vi "Periodic Tasks.vi"(8 "error in":errorcluster) -> ()   [LabVIEW 2017]
doc: "This VI runs in parallel to other robot code. It can contain as many user-defined periodic loops as you need. These can carry out PID or other sorts of timed response."
uses:
  <vilib>/Rock Robotics/WPI/Utilities/WPI_GetSetVariantRefNum.vi
  Robot Global Data.vi
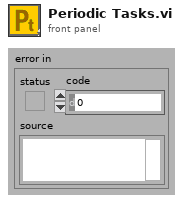
[diagram p1: front panel]
types:
  T1 = typedef "WPI_JoystickDevRef.ctl" = cluster{"Device":T2}
  T2 = typedef "WPI_JoystickDeviceEnum.ctl" = enum16{"USB 0", "USB 1", "USB 2", "USB 3", "USB 4", "USB 5"}
  T3 = typedef "WPI_SwitchDevRef.ctl" = cluster{"DevStatus":errorcluster, "DIO Channel":T4, "CntIndex":T5, "Normally Closed":bool}
  T4 = typedef "FPGA_DIOChannel.ctl" = enum8{"DIO 0", "DIO 1", "DIO 2", "DIO 3", "DIO 4", "DIO 5", "DIO 6", "DIO 7", "DIO 8", "DIO 9", "DIO MXP 0", "DIO MXP 1", "DIO MXP 2", "DIO MXP 3", "DIO MXP 4", "DIO MXP 5", "DIO MXP 6", "DIO MXP 7", "DIO MXP 8", "DIO MXP 9", "DIO MXP 10", "DIO MXP 11", "DIO MXP 12", "DIO MXP 13", "DIO MXP 14", "DIO MXP 15", "SPI Port CS1", "SPI Port CS2", "SPI Port CS3", "SPI Port MISO", "SPI Port MOSI", "Invalid"}
  T5 = typedef "FPGA_CounterCtrSystemIndex.ctl" = enum8{"Ctr 0", "Ctr 1", "Ctr 2", "Ctr 3", "Ctr 4", "Ctr 5", "Ctr 6", "Ctr 7", "Invalid"}
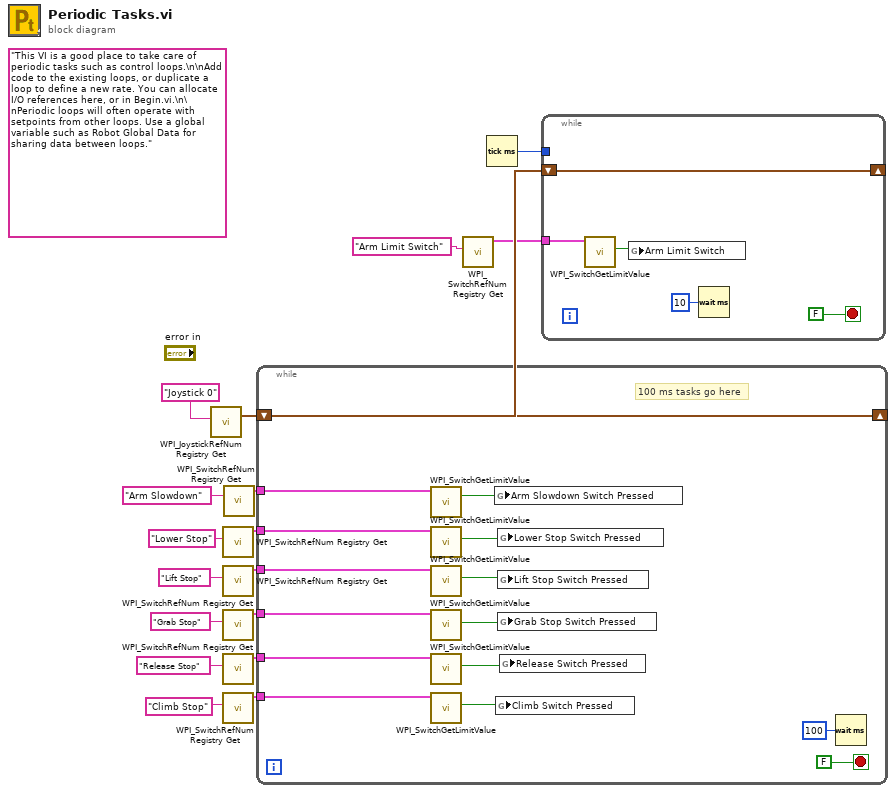
[diagram p0: block diagram]
diagram:
  (unwired) "This VI is a good place to take care of periodic tasks such as control loops.\n\nAdd code to the existing loops, or duplicate a loop to define a new rate. You can allocate I/O references here, or in Begin.vi.\n\nPeriodic loops will often operate with setpoints from other loops. Use a global variable such as Robot Global Data for sharing data between loops."
  n1 = call <vilib>:"WPI_JoystickRefNum Registry Get.vi"("refnum name"="Joystick 0") -> ("JoystickDevRef"=w16:T1)  [unwired: 1 in, 9 out]
  n2 = call <vilib>:"WPI_SwitchRefNum Registry Get.vi"("refnum name"="Lower Stop") -> ("SwitchDevRef"=w7:T3)  [unwired: 9 in, 1 out]
  n3 = call <vilib>:"WPI_SwitchRefNum Registry Get.vi"("refnum name"="Lift Stop") -> ("SwitchDevRef"=w6:T3)  [unwired: 9 in, 1 out]
  n4 = call <vilib>:"WPI_SwitchRefNum Registry Get.vi"("refnum name"="Grab Stop") -> ("SwitchDevRef"=w5:T3)  [unwired: 9 in, 1 out]
  n5 = call <vilib>:"WPI_SwitchRefNum Registry Get.vi"("refnum name"="Release Stop") -> ("SwitchDevRef"=w4:T3)  [unwired: 9 in, 1 out]
  n6 = call <vilib>:"WPI_SwitchRefNum Registry Get.vi"("refnum name"="Climb Stop") -> ("SwitchDevRef"=w3:T3)  [unwired: 9 in, 1 out]
  n7 = call <vilib>:"WPI_SwitchRefNum Registry Get.vi"("refnum name"="Arm Slowdown") -> ("SwitchDevRef"=w13:T3)  [unwired: 9 in, 1 out]
  n8 = while {
    shift-right: [w30] -> _
    shift-left: w16 -> [w30]
    tunnel: w13 -> [w29]
    tunnel: w7 -> [w27]
    tunnel: w6 -> [w26]
    tunnel: w5 -> [w25]
    tunnel: w4 -> [w24]
    tunnel: w3 -> [w23]
    stop <- FALSE stop-if-true
    # "100 ms tasks go here"
    n9 = call <vilib>:"WPI_SwitchGetLimitValue.vi"("SwitchDevRef"=w29) -> ("Switch Pressed"=w28:bool)  [unwired: 8 in, 2 out]
    n10 = call <vilib>:"WPI_SwitchGetLimitValue.vi"("SwitchDevRef"=w27) -> ("Switch Pressed"=w22:bool)  [unwired: 8 in, 2 out]
    n11 = call <vilib>:"WPI_SwitchGetLimitValue.vi"("SwitchDevRef"=w26) -> ("Switch Pressed"=w21:bool)  [unwired: 8 in, 2 out]
    n12 = call <vilib>:"WPI_SwitchGetLimitValue.vi"("SwitchDevRef"=w25) -> ("Switch Pressed"=w20:bool)  [unwired: 8 in, 2 out]
    n13 = call <vilib>:"WPI_SwitchGetLimitValue.vi"("SwitchDevRef"=w24) -> ("Switch Pressed"=w19:bool)  [unwired: 8 in, 2 out]
    n14 = call <vilib>:"WPI_SwitchGetLimitValue.vi"("SwitchDevRef"=w23) -> ("Switch Pressed"=w18:bool)  [unwired: 8 in, 2 out]
    n15 = global write "Robot Global Data.vi" "Arm Slowdown Switch Pressed"(w28) -> ()
    n16 = global write "Robot Global Data.vi" "Climb Switch Pressed"(w18) -> ()
    n17 = global write "Robot Global Data.vi" "Lower Stop Switch Pressed"(w22) -> ()
    n18 = global write "Robot Global Data.vi" "Lift Stop Switch Pressed"(w21) -> ()
    n19 = global write "Robot Global Data.vi" "Grab Stop Switch Pressed"(w20) -> ()
    n20 = global write "Robot Global Data.vi" "Release Switch Pressed"(w19) -> ()
    n21 = Wait (ms)(milliseconds to wait=u32 100) -> ()  [unwired: 1 out]
  }
  n22 = call <vilib>:"WPI_SwitchRefNum Registry Get.vi"("refnum name"="Arm Limit Switch") -> ("SwitchDevRef"=w1:T3)  [unwired: 9 in, 1 out]
  n23 = Tick Count (ms)() -> (millisecond timer value=w15:u32)
  n24 = while {
    shift-right: [w36] -> _
    shift-left: w16 -> [w36]
    tunnel: w15 -> [_]
    tunnel: w1 -> [w34]
    stop <- FALSE stop-if-true
    n25 = call <vilib>:"WPI_SwitchGetLimitValue.vi"("SwitchDevRef"=w34) -> ("Switch Pressed"=w33:bool)  [unwired: 8 in, 2 out]
    n26 = global write "Robot Global Data.vi" "Arm Limit Switch"(w33) -> ()
    n27 = Wait (ms)(milliseconds to wait=u32 10) -> ()  [unwired: 1 out]
  }
